vi "multi-function-fpga-TMP.vi"() -> ()   [LabVIEW 2016]
uses:
  fpga Control.ctl
  <vilib>/rvi/Emulation/niFpgaGetClockAttributes.vi
  <vilib>/rvi/Emulation/niFpgaSctlEmulationGetInTimedLoop.vi
  <vilib>/rvi/Emulation/niFpgaEmulationReportErrorSimple.vi
  <vilib>/rvi/Emulation/niFpgaProcessEmulError.vi
  <vilib>/rvi/Emulation/niFpgaCriticalErrorInLSC.vi
  <vilib>/rvi/eio/common/nirviEmuTemplateMethod_errors.vi
  <vilib>/eio/EIONode/EIONode.xnode
panel:
  in  "Update":bool
  in  "fpga controls":T1[](array[typedef]) {"Output - HI" format="%#_17g"; "Output - LO" format="%#_17g"; "Input - B" items=["DIO0", "DIO1", "DIO2", "DIO3", "DIO4", "DIO5", "DIO6", "DIO7", "DIO8", "DIO9", "DIO10", "DIO11", "DIO12", "DIO13", "DIO14", "DIO15", "DIO16", "DIO17", "DIO18", "DIO19", "DIO20", "DIO21", "DIO22", "DIO23", "DIO24", "DIO25", "DIO26", "DIO27", "DIO28", "DIO29", "DIO30", "DIO31"]; "Input - A" items=["DIO0", "DIO1", "DIO2", "DIO3", "DIO4", "DIO5", "DIO6", "DIO7", "DIO8", "DIO9", "DIO10", "DIO11", "DIO12", "DIO13", "DIO14", "DIO15", "DIO16", "DIO17", "DIO18", "DIO19", "DIO20", "DIO21", "DIO22", "DIO23", "DIO24", "DIO25", "DIO26", "DIO27", "DIO28", "DIO29", "DIO30", "DIO31"]; "Step Size" format="%#_17g"; "Begin" format="%#_17g"; "Operation" items=["OFF", "SWITCH", "AND GATE", "OR GATE", "ITERATION"]}
  in  "shutdown":bool
  # "Boolean Operation Outputs"
  # "Iteration Operation Outputs"
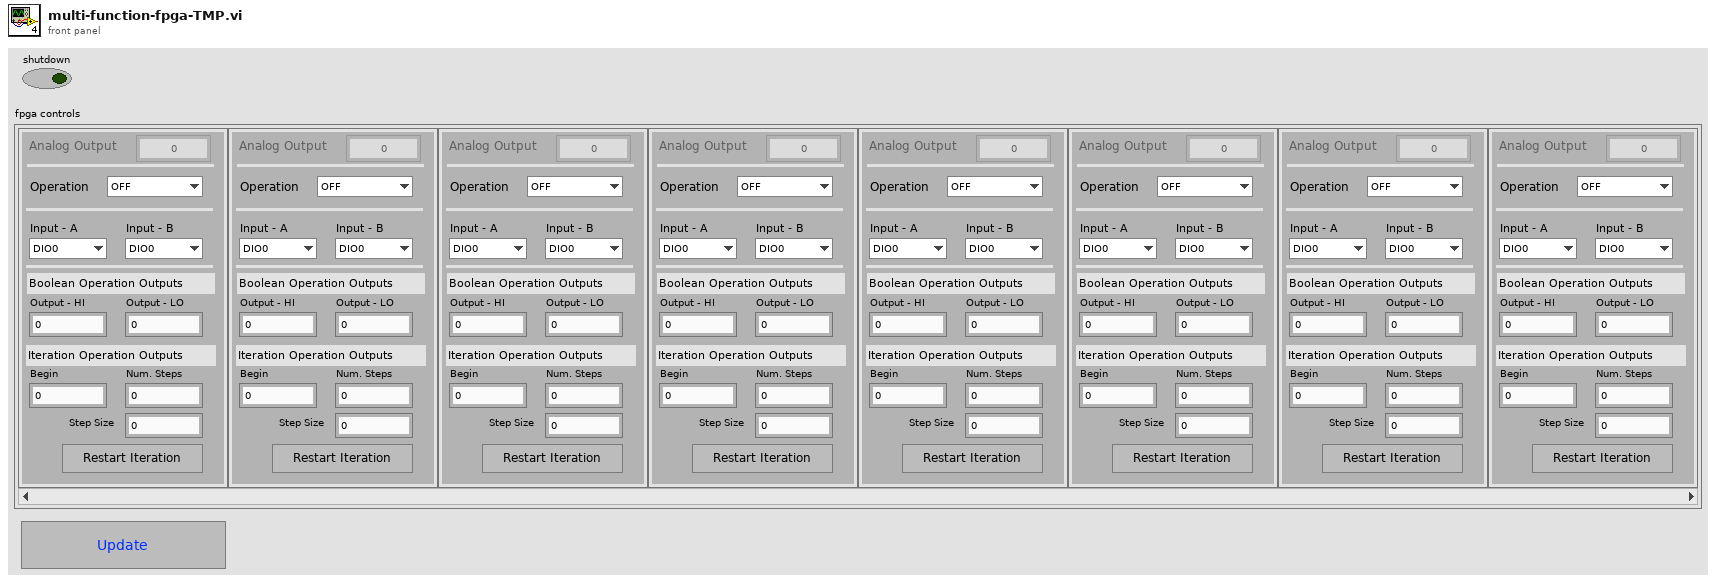
[diagram p1: front panel]
types:
  T1 = typedef "fpga Control.ctl" = cluster{"Operation":i16, "Num. Steps":u16, "Begin":sgl, "Step Size":sgl, "Input - A":i16, "Input - B":i16, "Output - LO":sgl, "Output - HI":sgl, "Reset":bool, "Analog Output":i16}
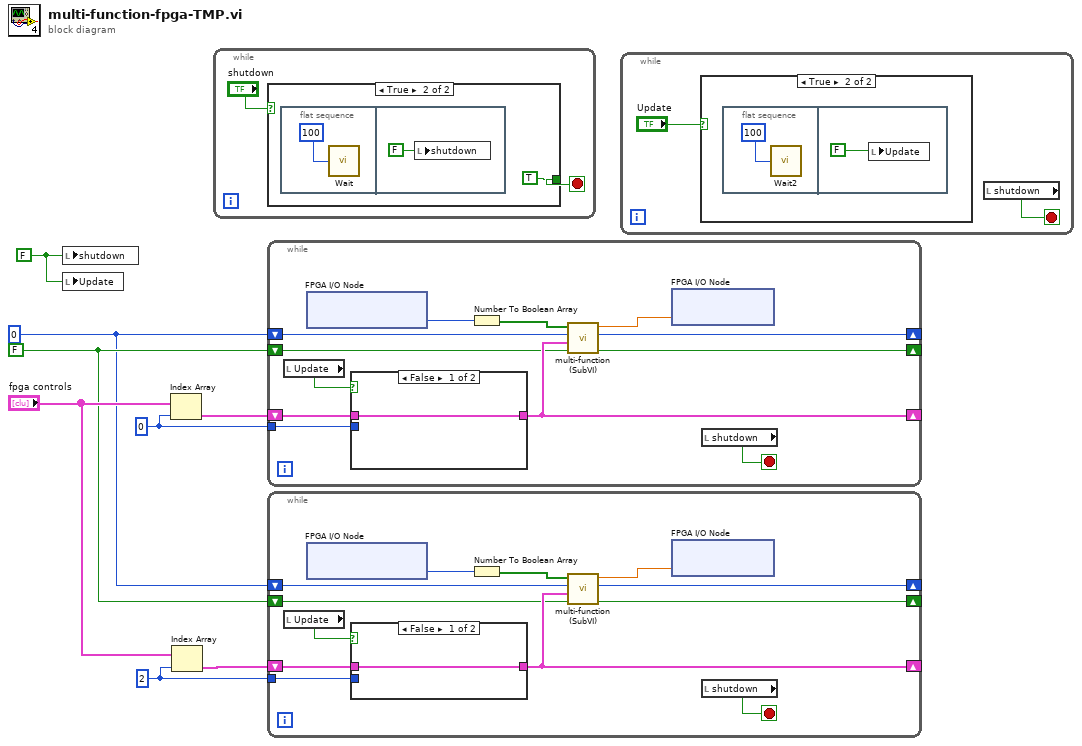
[diagram p0: block diagram]
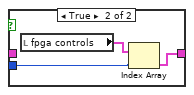
[diagram p2: hidden frame]
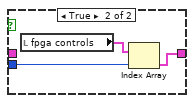
[diagram p5: hidden frame]
diagram:
  w3 = 2 ("index")
  w7 = FALSE ("parallel_shutodwn")
  w2 = FALSE
  w6 = 0 ("index")
  w1 = u16 0 ("Iter Num In")
  n1 = local write "shutdown"(w7) -> ()
  n2 = local write "Update"(w7) -> ()
  n3 = Index Array(array="fpga controls", index=w6) -> (element=w8:T1)
  n4 = Index Array(array="fpga controls", index=w3) -> (element=w5:T1)
  n5 = while {
    stop <- w9 stop-if-true
    n6 = case shown="True" "shutdown" {
      selector: "shutdown" -> [w11 _]
      tunnel: [w11 TRUE] -> w9
      frame False {
      }
      frame True {
        n7 = flat-sequence {
          frame #0 {
            n8 = call "Wait"("Count(mSec)"=u32 100) -> ()  [unwired: 1 out]
          }
          frame #1 {
            n9 = local write "shutdown"(FALSE ("parallel_shutodwn")) -> ()
          }
        }
      }
    }
  }
  n10 = while {
    shift-right: [w17] -> _
    shift-left: w1 -> [w24]
    shift-right: [w21] -> _
    shift-left: w8 -> [w22]
    shift-right: [w16] -> _
    shift-left: w2 -> [w20]
    tunnel: w6 -> [w15]
    stop <- w18 stop-if-true
    n11 = local read "Update"() -> (w23:bool)
    n12 = xnode "FPGA I/O Node"() -> ("Mod2/DIO31:0"=w26:u32)  [unwired: 1 in, 1 out]
    n13 = case shown="False" w23 {
      tunnel: w22 -> [w27 _]
      tunnel: [w27 w30] -> w21
      tunnel: w15 -> [_ w28]
      frame False {
      }
      frame True {
        n14 = local read "fpga controls"() -> (w29:T1[])
        n15 = Index Array(array=w29, index=w28) -> (element=w30:T1)
      }
    }
    n16 = Number To Boolean Array(number=w26) -> (Boolean array=w25:bool[])
    n17 = call "multi-function (SubVI).vi"("Step Value Flag In"=w20, "Channel"=w21, "Iter Num In"=w24, "Array"=w25) -> ("Step Value Flag Out"=w16:bool, "Iter Num Out"=w17:u16, "AO out"=w19:sgl)  [unwired: 5 in]
    n18 = xnode "FPGA I/O Node"("Mod4/AO0"=w19) -> ()  [unwired: 1 in, 1 out]
    n19 = local read "shutdown"() -> (w18:bool)
  }
  n20 = while {
    shift-right: [w33] -> _
    shift-left: w1 -> [w40]
    shift-right: [w37] -> _
    shift-left: w5 -> [w38]
    shift-right: [w32] -> _
    shift-left: w2 -> [w36]
    tunnel: w3 -> [w31]
    stop <- w34 stop-if-true
    n21 = local read "Update"() -> (w39:bool)
    n22 = xnode "FPGA I/O Node"() -> ("Mod2/DIO31:0"=w42:u32)  [unwired: 1 in, 1 out]
    n23 = case shown="False" w39 {
      tunnel: w38 -> [w43 _]
      tunnel: [w43 w46] -> w37
      tunnel: w31 -> [_ w44]
      frame False {
      }
      frame True {
        n24 = local read "fpga controls"() -> (w45:T1[])
        n25 = Index Array(array=w45, index=w44) -> (element=w46:T1)
      }
    }
    n26 = Number To Boolean Array(number=w42) -> (Boolean array=w41:bool[])
    n27 = call "multi-function (SubVI).vi"("Step Value Flag In"=w36, "Channel"=w37, "Iter Num In"=w40, "Array"=w41) -> ("Step Value Flag Out"=w32:bool, "Iter Num Out"=w33:u16, "AO out"=w35:sgl)  [unwired: 5 in]
    n28 = xnode "FPGA I/O Node"("Mod4/AO1"=w35) -> ()  [unwired: 1 in, 1 out]
    n29 = local read "shutdown"() -> (w34:bool)
  }
  n30 = while {
    stop <- w47 stop-if-true
    n31 = case shown="True" "Update" {
      frame False {
      }
      frame True {
        n32 = flat-sequence {
          frame #0 {
            n33 = call "Wait2"("Count(mSec)"=u32 100) -> ()  [unwired: 1 out]
          }
          frame #1 {
            n34 = local write "Update"(FALSE ("parallel_shutodwn")) -> ()
          }
        }
      }
    }
    n35 = local read "shutdown"() -> (w47:bool)
  }
